vi "Update Action History.vi"(8 "error in (no error)":errorcluster, 10 "Action":string, 11 "Tamer in":refnum<class "Tamer.lvclass">) -> (0 "error out":errorcluster, 3 "Tamer out":refnum<class "Tamer.lvclass">)   [LabVIEW 2020, in "Tamer.lvlib" / "Tamer.lvclass"]
uses:
  Tamer.lvclass
  C:/Users/marco/Documents/GitHub_Lab/TALOS/talos/Father of all uServices/Father of all uServices/Father of all uServices.lvclass
  Tamer.lvclass/Tamer.ctl
  Classes/Log/Log.lvclass/Log.ctl
  Ancestor/Ancestor/Ancestor.lvclass/Ancestor.ctl
  Father of all uServices/Father of all uServices/Father of all uServices.lvclass/Father of all uServices.ctl
  Classes/Log/Write.vi
  Father of all uServices/Father of all uServices/Children Methods/Update GUI.vi
  Support VIs/Generate Error.vi
  FGV/Error Memory/Get Error Description.vi
  Support VIs/Get PC name.vi
  Ancestor/Ancestor/Read ID.vi
  Support VIs/Get Class Name.vi
  <vilib>/Utility/error.llb/Clear Errors.vi
  FGV/Error Memory/Error Memory Core.vi
  <vilib>/AdvancedString/Delimited String to 1D String Array.vi
  Support VIs/Circus Root Path.vi
  FGV/Error Memory/Error Crt Lvl checker.vi
  FGV/Error Memory/Error Memory Core.vi/40c8088d-b597-4017-91af-faa98e00292e.vi
  FGV/Error Memory/Error Memory Core.vi/d4a3ab98-063c-4e44-b43d-fbdcfe6c2be2.vi
  Classes/Log/Rotate.vi
  Support VIs/Global Memory.vi
  <vilib>/Utility/LVClass/Get LV Class Name.vi
  Support VIs/Is in Packed Library.vi
  Support VIs/TALOS Root path.vi
  Support VIs/Read CSV worksheet.vi
  Support VIs/Global Constants.vi
  <vilib>/Utility/error.llb/General Error Handler.vi
  Father of all uServices/Father of all uServices/Children Methods/Get GUI Item Value - String.vi
  Father of all uServices/Father of all uServices/Multiline string updater.vi
  Support VIs/Error Log.vi
  Ancestor/Ancestor/Ancestor.lvclass
  <vilib>/Comparison/Equal/Equal Functor/Equal Functor.lvclass
  Classes/Log/Log.lvclass
  Father of all uServices/Father of all uServices/Father of all uServices.lvclass
  TALOS.lvlib
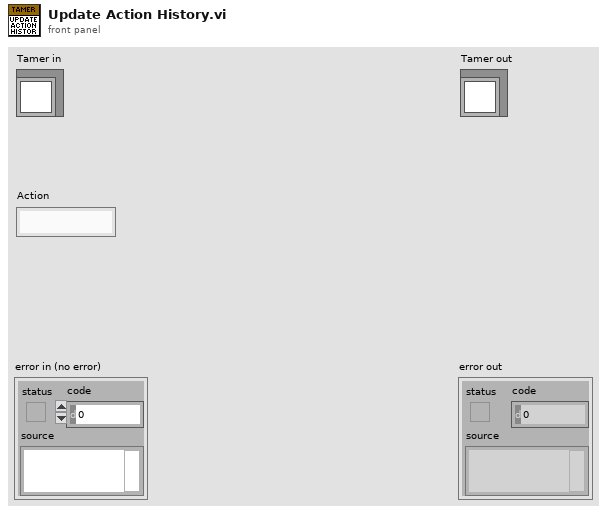
[diagram p1: front panel]
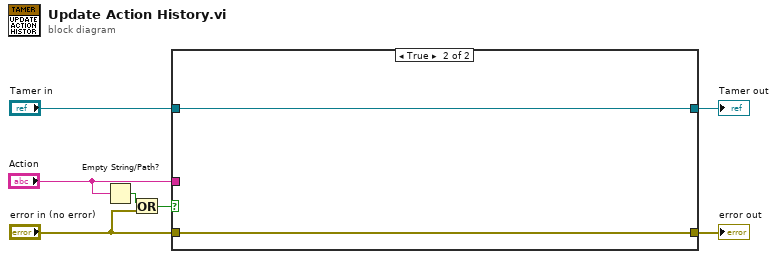
[diagram p0: block diagram]
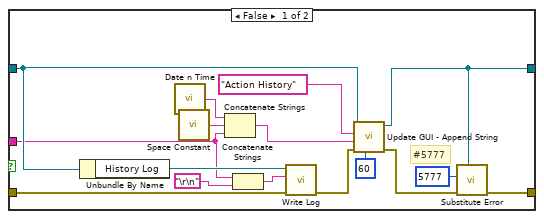
[diagram p2: hidden frame]
diagram:
  n1 = Empty String/Path?(string/path="Action") -> (empty?=w3:bool)
  n2 = Or(x=w3, y="error in (no error)") -> (x .or. y?=w1:bool)
  n3 = case shown="True" w1 {
    tunnel: [w10 w25] -> w7
    tunnel: [w9 w24] -> w5
    tunnel: "Tamer in" -> [w18 w24]
    tunnel: "Action" -> [w14 _]
    tunnel: "error in (no error)" -> [w13 w25]
    frame False {
      # "#5777"
      n4 = Unbundle By Name(w18) -> ("History Log"=w16:refnum<class "Log.lvclass">)
      n5 = call "Date n Time.vi"() -> ("Date & Time"=w21:string)  [unwired: 5 in]
      n6 = call <vilib>:"Space Constant.vi"() -> ("String"=w20:string)
      n7 = Concatenate Strings(w21, w20, w14) -> (w19:string)
      n8 = Concatenate Strings(w14, "\r\n") -> (w15:string)
      n9 = call "Write Log.vi"("error in (no error)"=w13, "Text"=w15, "Log in"=w16) -> ("error out"=w12:errorcluster)  [unwired: 7 in, 1 out]
      n10 = call "Update GUI - Append String.vi"("Lines to keep"=u8 60, "error in (no error)"=w12, "String"=w19, "GUI Item Name"="Action History", "Father of all uServices in"=w18) -> ("error out"=w11:errorcluster, "Father of all uServices out"=w9:refnum<class "Tamer.lvclass">)  [unwired: 5 in]
      n11 = call "Substitute Error.vi"("LabVIEW Object"=w9, "error in (no error)"=w11, "Error Code"=5777) -> ("error out"=w10:errorcluster)  [unwired: 8 in]
    }
    frame True {
    }
  }
  "error out" <- w7
  "Tamer out" <- w5
